vi "Unflatten From JSON String.vi"(6 "Nulls as Defaults (F)":bool, 7 "Type and Defaults":variant, 8 "error in (no error)":errorcluster, 11 "JSON String":string) -> (0 "error out":errorcluster, 3 "Variant":variant)   [LabVIEW 2015, in "JKI JSON Serialization.lvlib"]
doc: "Converts <b>JSON String</b> to <b>Variant</b>. If <b>Type and Defaults</b> is provided, converts JSON string to the specified type if the type is compatible with the value of the JSON String. For any cluster element in Type and Defaults, the value of the element in Type and Default is used if element with the same name is not present in the JSON String. If <b>Nulls as Defaults </b> is true, returns the default value as provided in Type and Defaults when null value is encountered in input tree."
uses:
  JKI JSON Serialization.lvlib
  Deserializer/JSON Deserializer/JSON Deserializer.lvclass
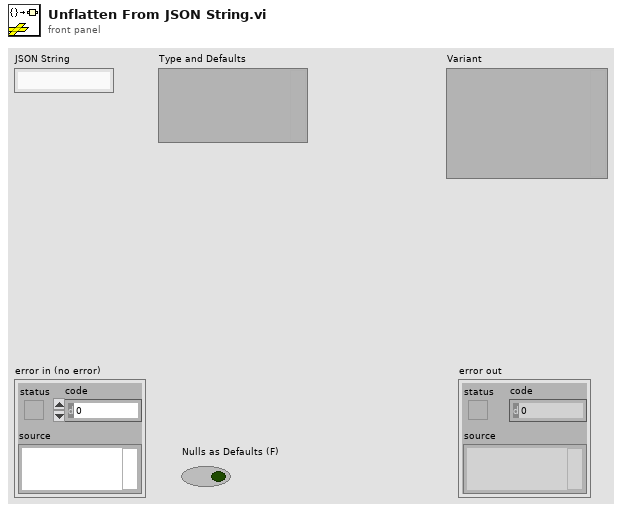
[diagram p1: front panel]
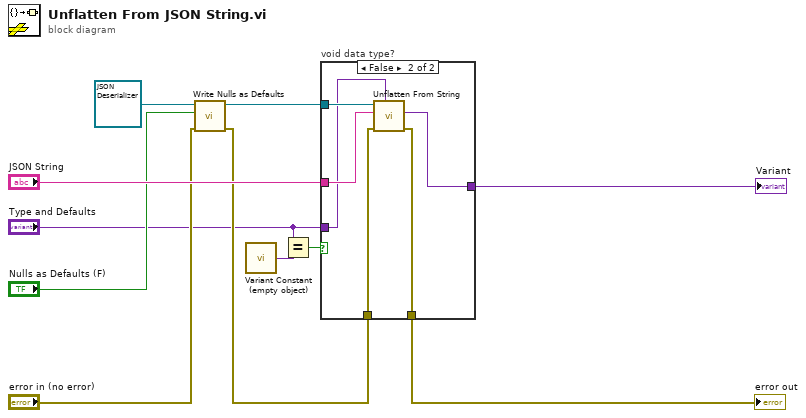
[diagram p0: block diagram]
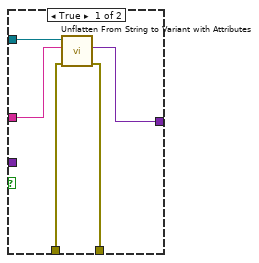
[diagram p2: hidden frame]
diagram:
  n1 = call-dynamic "Write Nulls as Defaults.vi"("error in (no error)"="error in (no error)", "Nulls as Defaults"="Nulls as Defaults (F)", "JSON Deserializer in"=refnum<class "JSON Deserializer.lvclass"> refnum ("Deserializer in")) -> ("error out"=w5:errorcluster, "JSON Deserializer out"=w7:refnum<class "JSON Deserializer.lvclass">)  [unwired: 7 in]
  n2 = call "Variant Constant (empty object).vi"() -> ("Empty Object"=w3:variant)  [unwired: 2 in]
  n3 = Equal?(x="Type and Defaults", y=w3) -> (x = y?=w1:bool)
  n4 = case "void data type?" shown="False" w1 {
    tunnel: "JSON String" -> [w16 w22]
    tunnel: [w15 w21] -> w10
    tunnel: [w14 w20] -> w9
    tunnel: w7 -> [w13 w19]
    tunnel: w5 -> [w12 w18]
    tunnel: "Type and Defaults" -> [_ w17]
    frame True {
      n5 = call-dynamic "Unflatten From String to Variant with Attributes.vi"("error in (no error)"=w12, "String"=w16, "Deserializer in"=w13) -> ("error out"=w15:errorcluster, "Variant with Attributes"=w14:variant)  [unwired: 6 in, 1 out]
    }
    frame False {
      n6 = call-dynamic "Unflatten From String.vi"("Type and Defaults"=w17, "error in (no error)"=w18, "String"=w22, "Deserializer in"=w19) -> ("error out"=w21:errorcluster, "Variant"=w20:variant)  [unwired: 5 in, 1 out]
    }
  }
  "error out" <- w10
  "Variant" <- w9
